vi "Connect-Disconnect.vi"(7 "Address":string, 8 "Error In":errorcluster) -> (0 "Error Out":errorcluster)   [LabVIEW 2018, in "Tests.lvlib" / "Session.lvlib"]
uses:
  Session.lvlib
  <vilib>/addons/_JKI Toolkits/Caraya/classes/Test/Test.lvclass
  src/Toolkit/SSH/SSH.lvclass
  src/Toolkit/Session/Session.lvclass
  <vilib>/addons/_JKI Toolkits/Caraya/classes/Assert/Assert.lvclass
  Tests.lvlib
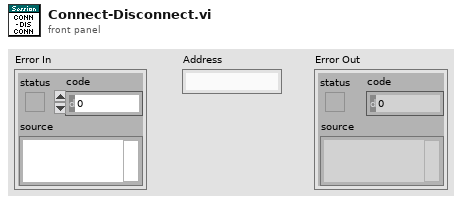
[diagram p1: front panel]
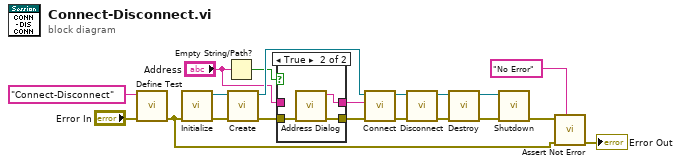
[diagram p0: block diagram]
diagram:
  n1 = call <vilib>:"Define Test.vi"("error in (no error)"="Error In", "Label (VI Title)"="Connect-Disconnect") -> ("error out"=w12:errorcluster)  [unwired: 9 in]
  n2 = call "Initialize.vi"("Error In"=w12) -> ("Error Out"=w18:errorcluster, "SSH"=w17:refnum<class "SSH.lvclass">)  [unwired: 9 in]
  n3 = Empty String/Path?(string/path="Address") -> (empty?=w5:bool)
  n4 = call "Create.vi"("Error In"=w18, "SSH"=w17) -> ("Error Out"=w2:errorcluster, "Sesssion"=w10:refnum<class "Session.lvclass">)  [unwired: 8 in]
  n5 = case shown="True" w5 {
    tunnel: w2 -> [w21 w25]
    tunnel: [w21 w24] -> w3
    tunnel: [w22 w23] -> w4
    tunnel: "Address" -> [w22 _]
    frame False {
    }
    frame True {
      n6 = call "Address Dialog.vi"("Error In"=w25) -> ("Error Out"=w24:errorcluster, "Address Out"=w23:string)  [unwired: 9 in]
    }
  }
  n7 = call "Connect.vi"("Error In"=w3, "Address"=w4, "Session In"=w10) -> ("Error Out"=w6:errorcluster, "Sesssion Out"=w7:refnum<class "Session.lvclass">)  [unwired: 7 in]
  n8 = call "Disconnect.vi"("Error In"=w6, "Session In"=w7) -> ("Error Out"=w8:errorcluster, "Sesssion Out"=w9:refnum<class "Session.lvclass">)  [unwired: 8 in]
  n9 = call "Destroy.vi"("Error In"=w8, "Session"=w9) -> ("Error Out"=w15:errorcluster, "SSH"=w16:refnum<class "SSH.lvclass">)  [unwired: 8 in]
  n10 = call "Shutdown.vi"("Error In"=w15, "SSH"=w16) -> ("Error Out"=w14:errorcluster)  [unwired: 9 in]
  n11 = call <vilib>:"Assert Not Error.vi"("Label"="No Error", "error in (no error)"=w12, "Not Error?"=w14) -> ("error out"=→"Error Out":errorcluster)  [unwired: 8 in]
